vi "Relays plus AC input.vi"() -> ()   [LabVIEW 2014]
panel:
  out "Channel 3 Approx. 240V?":bool
  out "Channel 2 Approx. 240V?":bool
  out "Channel 1 Approx. 240V?":bool
  out "Phase C":dbl
  out "Phase B":dbl
  out "Phase A":dbl
  out "Waveform Graph":dynamicdata(graph) caption="Parallel Circuit Pk-Pk Supply Voltage (Chroma)"
  in  "stop":bool
  in  "?":bool
  in  "CH1":bool
  in  "CH3":bool
  in  "CH4":bool
  in  "CH1":bool
  in  "CH2":bool
  in  "CH3":bool
  in  "CH4":bool
  in  "CH1":bool
  in  "CH2":bool
  in  "CH3":bool
  in  "CH4":bool
  in  "CH1":bool
  in  "CH2":bool
  in  "CH3":bool
  in  "CH4":bool
  in  "CH1":bool
  in  "CH2":bool
  in  "CH2":bool
  in  "CH3":bool
  in  "CH4":bool
  in  "CH1":bool
  in  "CH2":bool
  in  "CH3":bool
  in  "CH4":bool
  in  "CH1":bool
  in  "CH2":bool
  in  "CH3":bool
  in  "CH4":bool
  in  "CH1":bool
  in  "CH2":bool
  in  "CH3":bool
  in  "CH4":bool
  in  "CH5":bool
  in  "CH6":bool
  in  "CH7":bool
  in  "CH8":bool
  in  "CH1":bool
  in  "CH2":bool
  in  "CH3":bool
  in  "CH4":bool
  in  "CH5":bool
  in  "CH6":bool
  in  "CH7":bool
  in  "CH8":bool
  # "cDAQ-9179 - 14 SLOT USB CHASSIS"
  # "MODULE 1"
  # "MODULE 2"
  # "MODULE 3"
  # "MODULE 4"
  # "MODULE 5"
  # "MODULE 6"
  # "MODULE 7"
  # "RL1     RL2      RL3    RL4"
  # "RL5     RL6     RL7     RL8"
  # "RL9    RL10    RL11  RL12"
  # "RL13   RL14   RL15  RL16"
  # "RL17   RL18   RL19  RL20  RL21"
  # "RL21   RL22   RL23   RL24"
  # "RL25   RL26   RL27  RL28"
  # "EXPORT\nCat     Cat    \n1-5        6"
  # "CAT3   \n   E2/\n   E1"
  # "AP1  Bat1\n v1.5\n90531"
  # "AP2     Bat2\n v4.5\n50059"
  # "AP3    Bat3\n v5.0\n50143"
  # "RL1   Bat4\n v1.5\n 819"
  # "RL2     Bat5\n v4.5\n 851"
  # "RL3   Mic\n v5.0   AP\n 006"
  # "Series\n/Para\n/Skt1"
  # "IHDs\n Skt2"
  # "Series Cct on/off\n3Ph    Ph1    Ph3"
  # "SIQ/ ESCC/\n             Auto-Disconnect"
  # "TAMPER:\n    DELV\n 1Ph    3Ph"
  # "UIQ-\n QA"
  # "MODULE 11"
  # "MODULE 12"
  # "RL40   RL41   RL42    RL43   RL44    RL45    RL46  RL47"
  # "RL48   RL49   RL50    RL51   RL52    RL53    RL54  RL55"
  # "TAMPER:         BOOST:            \nETBC Front        LC   LC           \n          cover     close open"
  # "RTC\n  2v/\n  0v"
  # "RTC     \nCat3   Cat3   Cat1\n v2        v3       v2"
  # "RTC                \nCat1      \n v3"
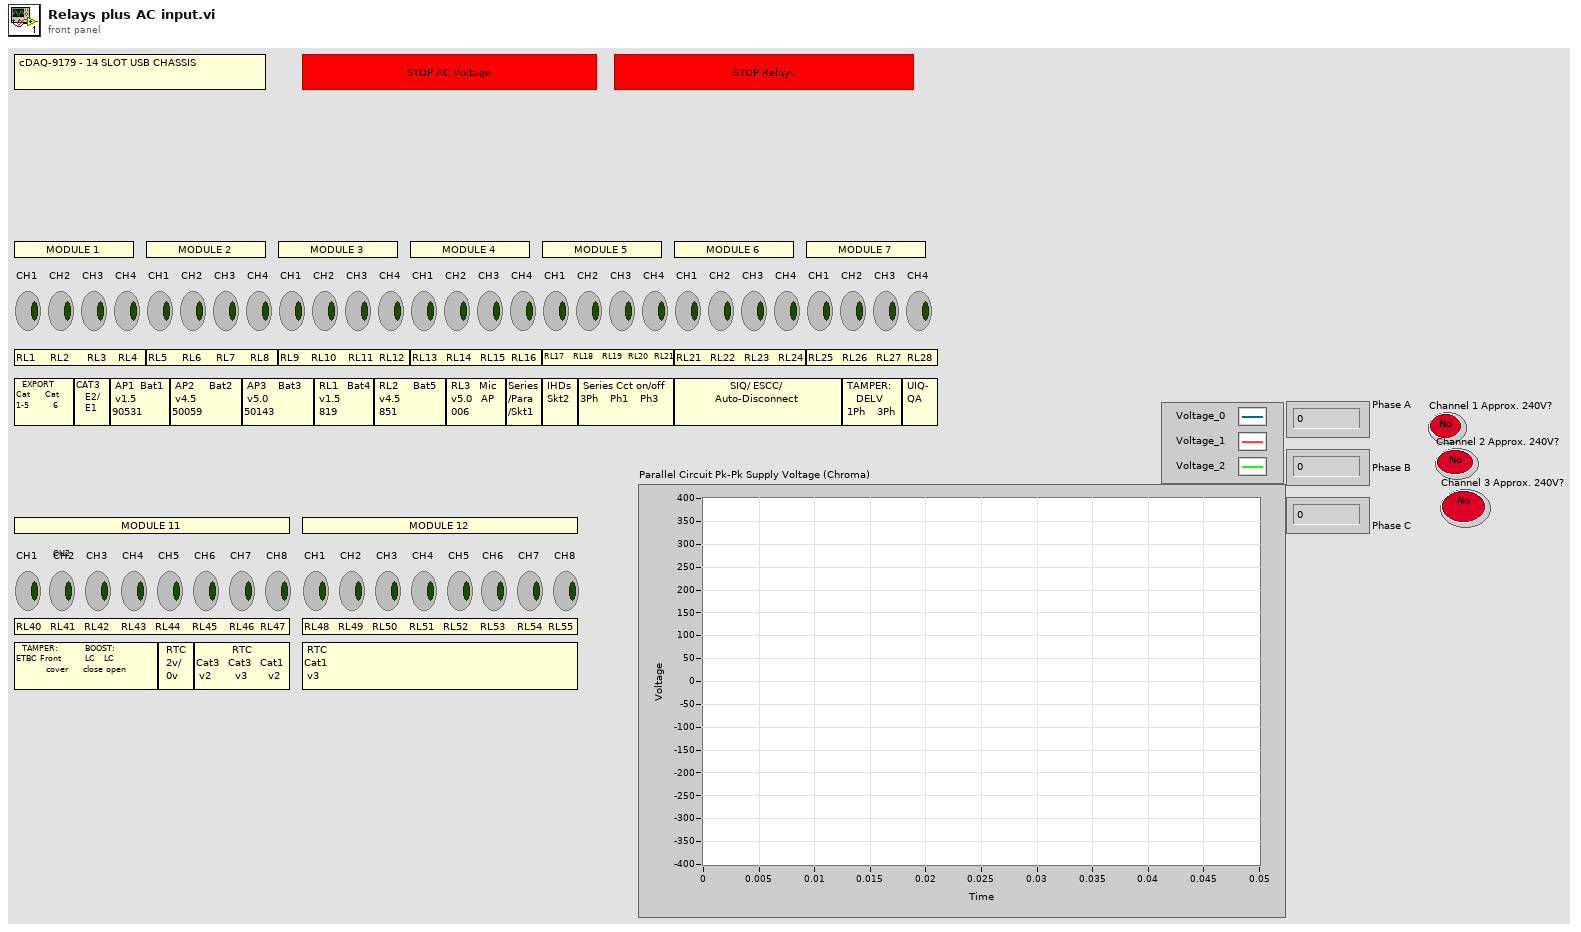
[diagram p1: front panel]
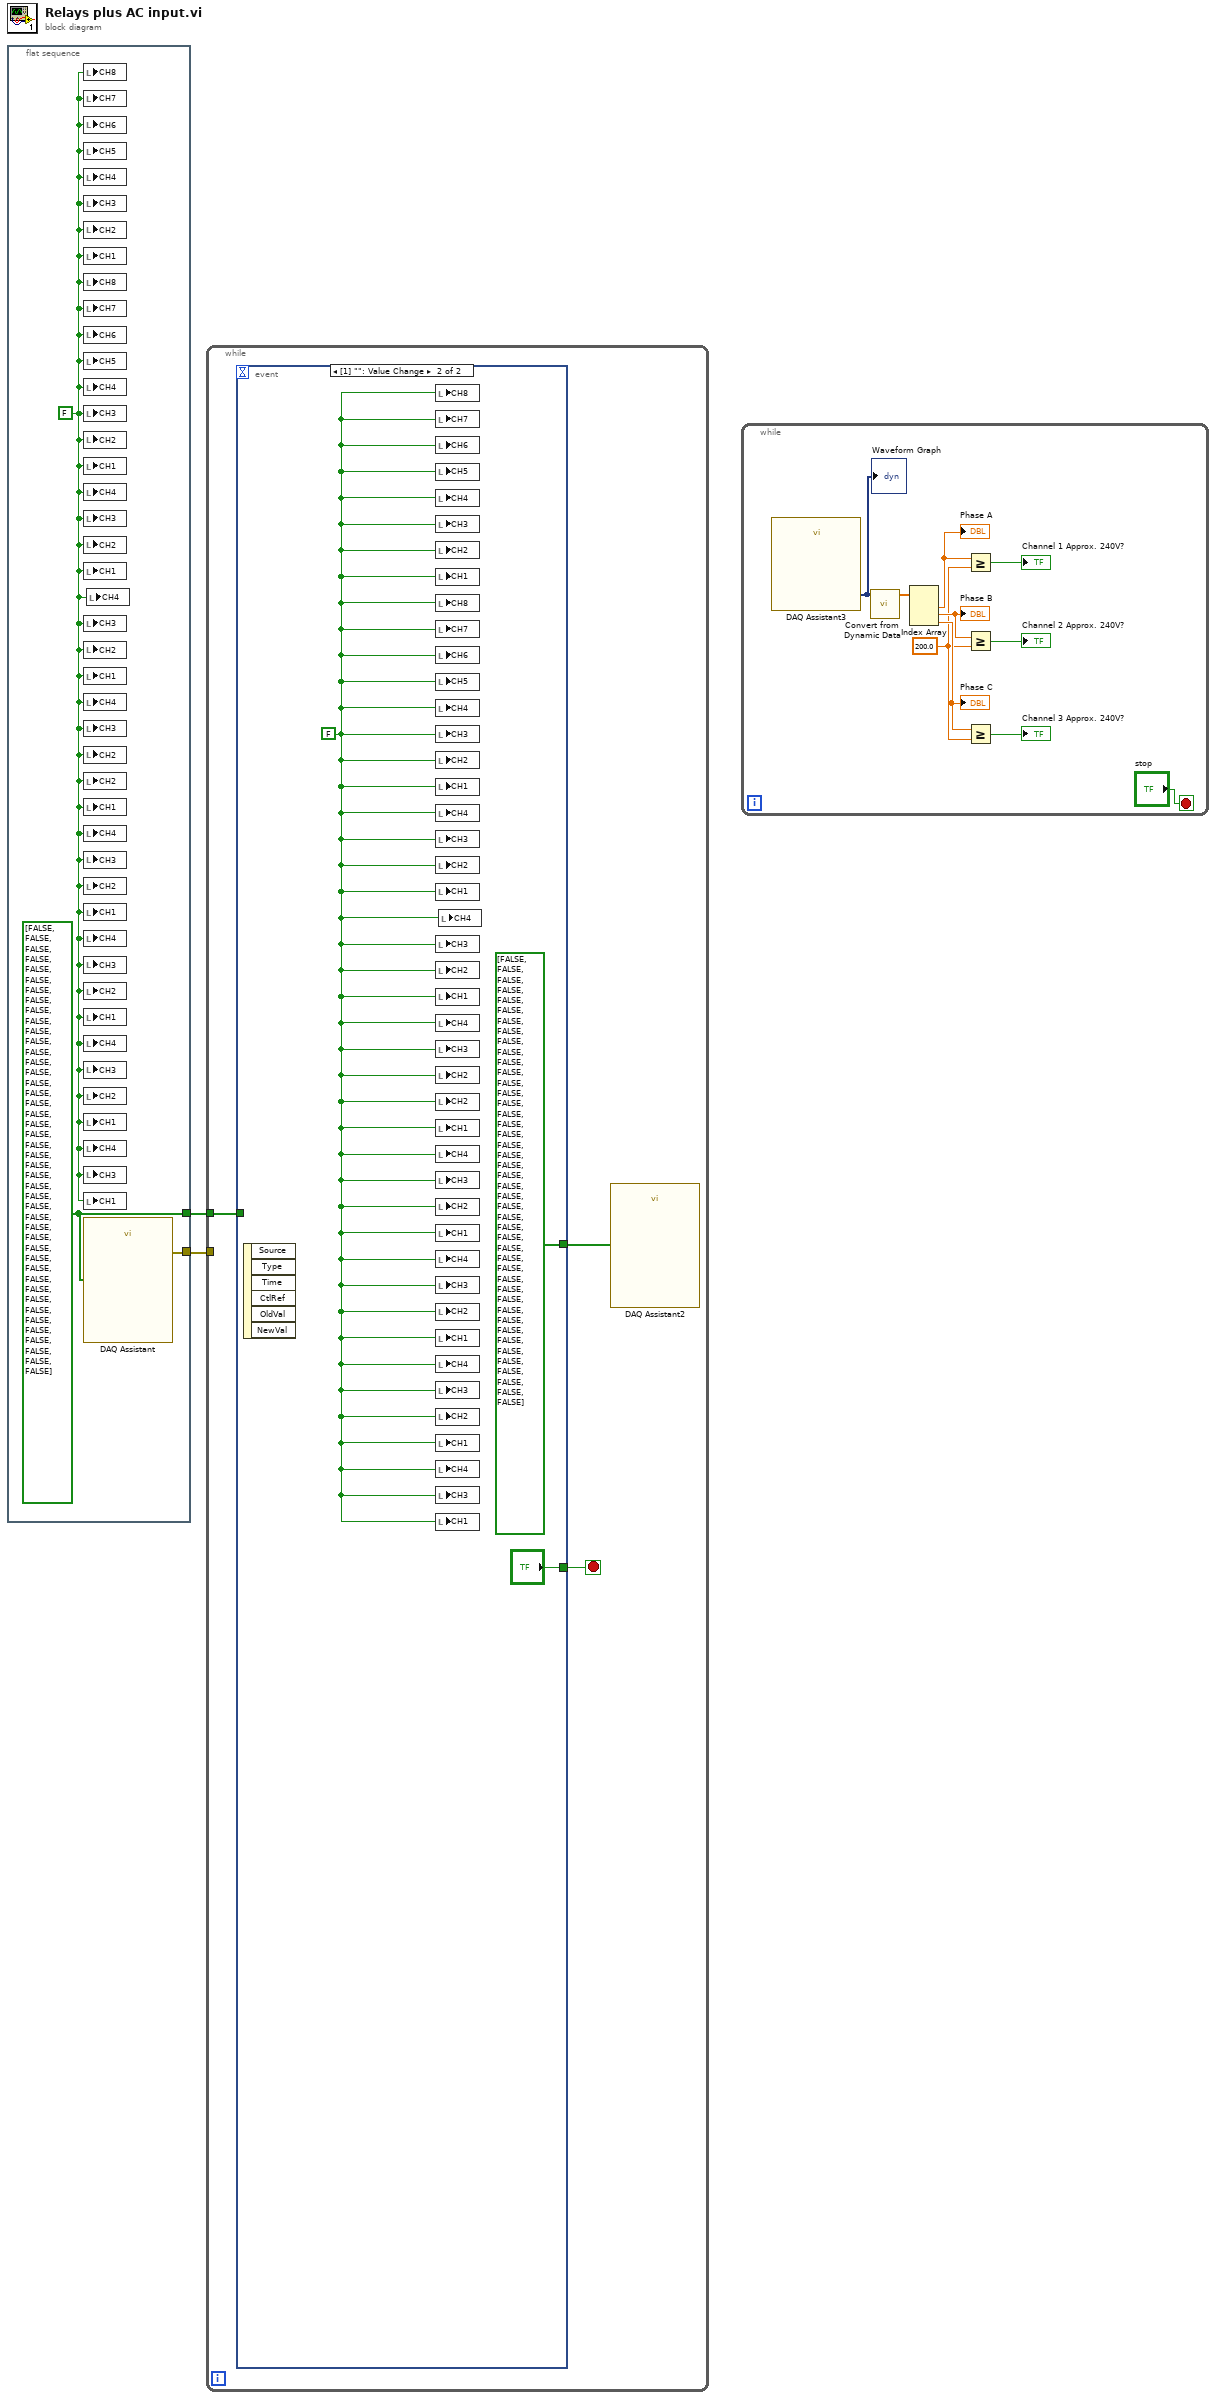
[diagram p0: block diagram]
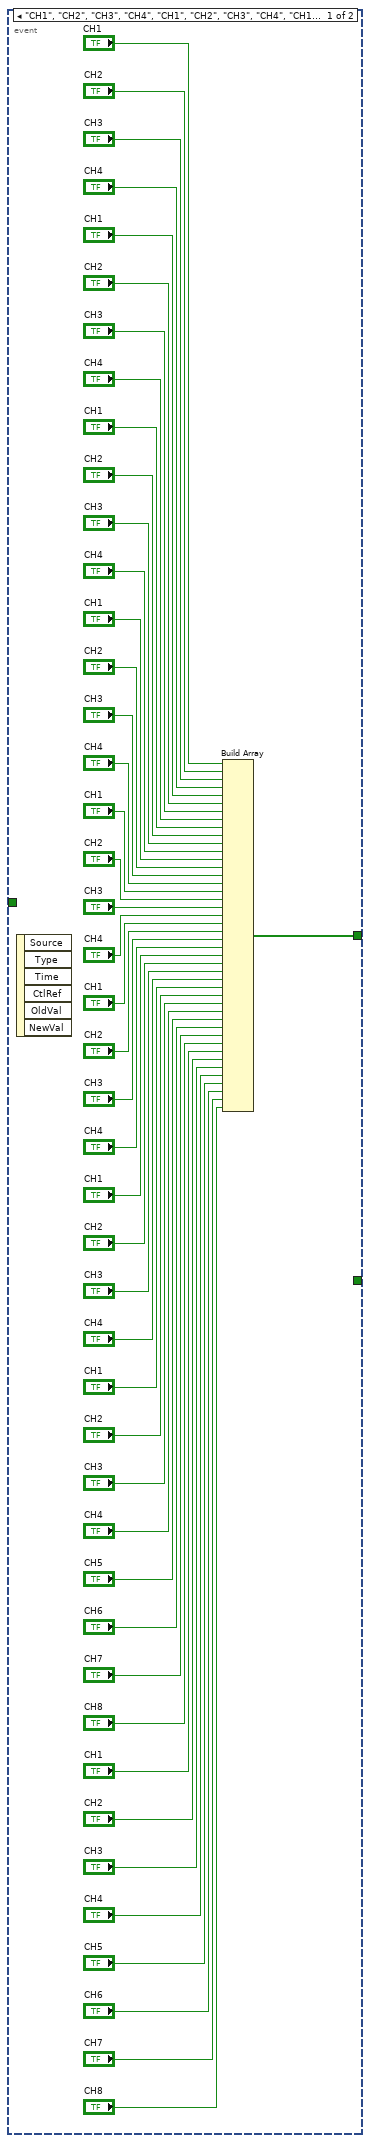
[diagram p2: hidden frame]
diagram:
  n1 = flat-sequence {
    tunnel: [w5] -> w2
    tunnel: [w4] -> w1
    frame #0 {
      w3 = FALSE
      w4 = bool[] [FALSE, FALSE, FALSE, FALSE, FALSE, FALSE, FALSE, FALSE, FALSE, FALSE, FALSE, FALSE, FALSE, FALSE, FALSE, FALSE, FALSE, FALSE, FALSE, FALSE, FALSE, FALSE, FALSE, FALSE, FALSE, FALSE, FALSE, FALSE, FALSE, FALSE, FALSE, FALSE, FALSE, FALSE, FALSE, FALSE, FALSE, FALSE, FALSE, FALSE, FALSE, FALSE, FALSE, FALSE]
      n2 = local write "CH8"(w3) -> ()
      n3 = local write "CH7"(w3) -> ()
      n4 = local write "CH6"(w3) -> ()
      n5 = local write "CH5"(w3) -> ()
      n6 = local write "CH4"(w3) -> ()
      n7 = local write "CH3"(w3) -> ()
      n8 = local write "CH2"(w3) -> ()
      n9 = local write "CH1"(w3) -> ()
      n10 = local write "CH8"(w3) -> ()
      n11 = local write "CH7"(w3) -> ()
      n12 = local write "CH6"(w3) -> ()
      n13 = local write "CH5"(w3) -> ()
      n14 = local write "CH4"(w3) -> ()
      n15 = local write "CH3"(w3) -> ()
      n16 = local write "CH2"(w3) -> ()
      n17 = local write "CH1"(w3) -> ()
      n18 = local write "CH4"(w3) -> ()
      n19 = local write "CH3"(w3) -> ()
      n20 = local write "CH2"(w3) -> ()
      n21 = local write "CH1"(w3) -> ()
      n22 = local write "CH3"(w3) -> ()
      n23 = local write "CH2"(w3) -> ()
      n24 = local write "CH1"(w3) -> ()
      n25 = local write "CH4"(w3) -> ()
      n26 = local write "CH3"(w3) -> ()
      n27 = local write "CH2"(w3) -> ()
      n28 = local write "CH2"(w3) -> ()
      n29 = local write "CH1"(w3) -> ()
      n30 = local write "CH4"(w3) -> ()
      n31 = local write "CH3"(w3) -> ()
      n32 = local write "CH2"(w3) -> ()
      n33 = local write "CH1"(w3) -> ()
      n34 = local write "CH4"(w3) -> ()
      n35 = local write "CH3"(w3) -> ()
      n36 = local write "CH2"(w3) -> ()
      n37 = local write "CH1"(w3) -> ()
      n38 = local write "CH4"(w3) -> ()
      n39 = local write "CH3"(w3) -> ()
      n40 = local write "CH2"(w3) -> ()
      n41 = local write "CH1"(w3) -> ()
      n42 = local write "CH4"(w3) -> ()
      n43 = local write "CH3"(w3) -> ()
      n44 = local write "CH1"(w3) -> ()
      n45 = call "DAQ Assistant"("data"=w4) -> ("error out"=w5:errorcluster)  [unwired: 17 in, 1 out]
      n46 = local write "CH4"(w3) -> ()
    }
  }
  n47 = while {
    tunnel: w2 -> [_]
    tunnel: w1 -> [w7]
    stop <- w8 stop-if-true
    n48 = event shown="[1] \"\": Value Change" {
      selector: _ -> [_ _]
      dyn-events: _ -> [_ _]
      timeout: _ -> [_ _]
      tunnel: [_ "?"] -> w8
      tunnel: w7 -> [_ _]
      tunnel: [w9 bool[] [FALSE, FALSE, FALSE, FALSE, FALSE, FALSE, FALSE, FALSE, FALSE, FALSE, FALSE, FALSE, FALSE, FALSE, FALSE, FALSE, FALSE, FALSE, FALSE, FALSE, FALSE, FALSE, FALSE, FALSE, FALSE, FALSE, FALSE, FALSE, FALSE, FALSE, FALSE, FALSE, FALSE, FALSE, FALSE, FALSE, FALSE, FALSE, FALSE, FALSE, FALSE, FALSE, FALSE, FALSE]] -> w6
      event "CH1", "CH2", "CH3", "CH4", "CH1", "CH2", "CH3", "CH4", "CH1", "CH2", "CH3", "CH4", "CH1", "CH2", "CH3", "CH4", "CH1", "CH2", "CH3", "CH4", "CH1", "CH2", "CH3", "CH4", "CH1", "CH2", "CH3", "CH4", "CH1", "CH2", "CH3", "CH4", "CH5", "CH6", "CH7", "CH8": Value Change {
        n49 = event-data() -> ()  [unwired: 1 in, 6 out]
        n50 = Build Array("CH1", "CH2", "CH3", "CH4", "CH1", "CH2", "CH3", "CH4", "CH1", "CH2", "CH3", "CH4", "CH1", "CH2", "CH3", "CH4", "CH1", "CH2", "CH3", "CH4", "CH1", "CH2", "CH3", "CH4", "CH1", "CH2", "CH3", "CH4", "CH1", "CH2", "CH3", "CH4", "CH5", "CH6", "CH7", "CH8", "CH1", "CH2", "CH3", "CH4", "CH5", "CH6", "CH7", "CH8") -> (w9:bool[])
      }
      event Value Change {
        w54 = FALSE
        n51 = event-data() -> ()  [unwired: 1 in, 6 out]
        n52 = local write "CH8"(w54) -> ()
        n53 = local write "CH7"(w54) -> ()
        n54 = local write "CH6"(w54) -> ()
        n55 = local write "CH5"(w54) -> ()
        n56 = local write "CH4"(w54) -> ()
        n57 = local write "CH3"(w54) -> ()
        n58 = local write "CH2"(w54) -> ()
        n59 = local write "CH1"(w54) -> ()
        n60 = local write "CH8"(w54) -> ()
        n61 = local write "CH7"(w54) -> ()
        n62 = local write "CH6"(w54) -> ()
        n63 = local write "CH5"(w54) -> ()
        n64 = local write "CH4"(w54) -> ()
        n65 = local write "CH3"(w54) -> ()
        n66 = local write "CH2"(w54) -> ()
        n67 = local write "CH1"(w54) -> ()
        n68 = local write "CH4"(w54) -> ()
        n69 = local write "CH3"(w54) -> ()
        n70 = local write "CH2"(w54) -> ()
        n71 = local write "CH1"(w54) -> ()
        n72 = local write "CH3"(w54) -> ()
        n73 = local write "CH2"(w54) -> ()
        n74 = local write "CH1"(w54) -> ()
        n75 = local write "CH4"(w54) -> ()
        n76 = local write "CH3"(w54) -> ()
        n77 = local write "CH2"(w54) -> ()
        n78 = local write "CH2"(w54) -> ()
        n79 = local write "CH1"(w54) -> ()
        n80 = local write "CH4"(w54) -> ()
        n81 = local write "CH3"(w54) -> ()
        n82 = local write "CH2"(w54) -> ()
        n83 = local write "CH1"(w54) -> ()
        n84 = local write "CH4"(w54) -> ()
        n85 = local write "CH3"(w54) -> ()
        n86 = local write "CH2"(w54) -> ()
        n87 = local write "CH1"(w54) -> ()
        n88 = local write "CH4"(w54) -> ()
        n89 = local write "CH3"(w54) -> ()
        n90 = local write "CH2"(w54) -> ()
        n91 = local write "CH1"(w54) -> ()
        n92 = local write "CH4"(w54) -> ()
        n93 = local write "CH3"(w54) -> ()
        n94 = local write "CH1"(w54) -> ()
        n95 = local write "CH4"(w54) -> ()
      }
    }
    n96 = call "DAQ Assistant2"("data"=w6) -> ()  [unwired: 17 in, 2 out]
  }
  n97 = while {
    stop <- "stop" stop-if-true
    w60 = 200.0 ("y")
    n98 = call "DAQ Assistant3"() -> ("data"=w65:dynamicdata)  [unwired: 17 in, 2 out]
    "Waveform Graph" <- w65
    n99 = call "Convert from Dynamic Data"("Dynamic Data Type"=w65) -> ("Array"=w64:dbl[])  [unwired: 3 in]
    n100 = Index Array(array=w64) -> (element #1=w63:dbl, element #2=w62:dbl, element #3=w61:dbl)  [unwired: 3 in]
    "Phase A" <- w63
    "Phase B" <- w62
    "Phase C" <- w61
    n101 = Greater Or Equal?(x=w63, y=w60) -> (x >= y?=→"Channel 1 Approx. 240V?":bool)
    n102 = Greater Or Equal?(x=w62, y=w60) -> (x >= y?=→"Channel 2 Approx. 240V?":bool)
    n103 = Greater Or Equal?(x=w61, y=w60) -> (x >= y?=→"Channel 3 Approx. 240V?":bool)
  }
